vi "Regenerate All Button Images.vi"(8 "error in (no error)":errorcluster, 11 "Display State In in":T1 caption="State") -> (0 "error out":errorcluster, 3 "Display State In out":T1 caption="State")   [LabVIEW 2018, in "Toolbar.xctl"]
doc: "Force the regeneration of all button images and caching thereore"
uses:
  Toolbar.xctl
  Button_Class/Button.lvclass
  Button_Class/Type Defs/Button Style.ctl
  Toolbar State.ctl
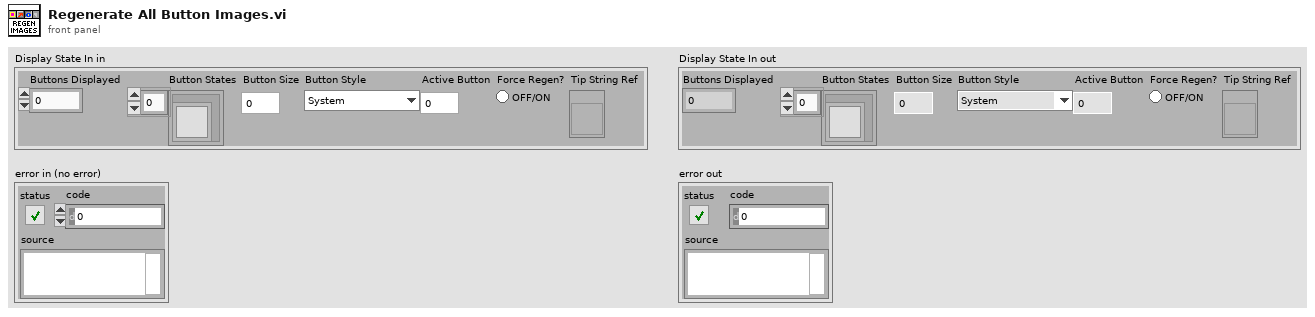
[diagram p1: front panel]
types:
  T1 = typedef "Toolbar.xctl/Toolbar State.ctl" = cluster{"Buttons Displayed":i32, "Button States":refnum<class "Button.lvclass">[], "Button Size":i32, "Button Style":T2, "Active Button":i32, "Force Regen?":bool, "Tip String Ref":refnum<vi>}
  T2 = typedef "Button.lvclass/Button Style.ctl" = enum16{"System", "Modern", "Classic", "Rounded", "Silver", "Ni Theme", "Metallic"}
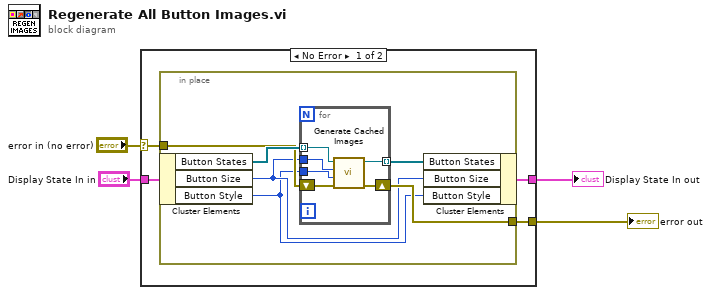
[diagram p0: block diagram]
diagram:
  n1 = case shown="No Error" "error in (no error)" {
    selector: "error in (no error)" -> [w6 w22]
    tunnel: [w8 w21] -> w4
    tunnel: [w7 w22] -> w3
    tunnel: "Display State In in" -> [w5 w21]
    frame No Error {
      n2 = in-place {
        in-place-border: w6 -> [w12]
        in-place-border: [w11] -> w7
        n3 = in-place-cluster #1(w5) -> ("Button States"=w13:refnum<class "Button.lvclass">[], "Button Size"=w10:i32, "Button Style"=w9:T2)
        n4 = for {
          tunnel: [w19] -> w14 mode=indexing
          tunnel: w13 -> [w20] mode=indexing
          tunnel: w10 -> [w18]
          tunnel: w9 -> [w17]
          shift-right: [w15] -> w11
          shift-left: w12 -> [w16]
          n5 = call-dynamic "Generate Cached Images.vi"("error in (no error)"=w16, "Button Style"=w17, "Button Size"=w18, "object in"=w20) -> ("error out"=w15:errorcluster, "object out"=w19:refnum<class "Button.lvclass">)  [unwired: 6 in]
        }
        n6 = in-place-cluster #1("Button States"=w14, "Button Size"=w10, "Button Style"=w9) -> (w8:T1)
      }
    }
    frame Error {
    }
  }
  "Display State In out" <- w4
  "error out" <- w3
